vi "Add Files.vi"(8 "error in (no error)":errorcluster, 9 "Results":map{path, string}(c390), 10 "Files":set{path}(c389), 11 "File Tree In":refnum<class "File Tree.lvclass">) -> (0 "error out":errorcluster, 3 "File Tree Out":refnum<class "File Tree.lvclass">)   [LabVIEW 2020, in "File Tree.lvclass"]
uses:
  File Tree.lvclass
  File Tree.lvclass/File Tree.ctl
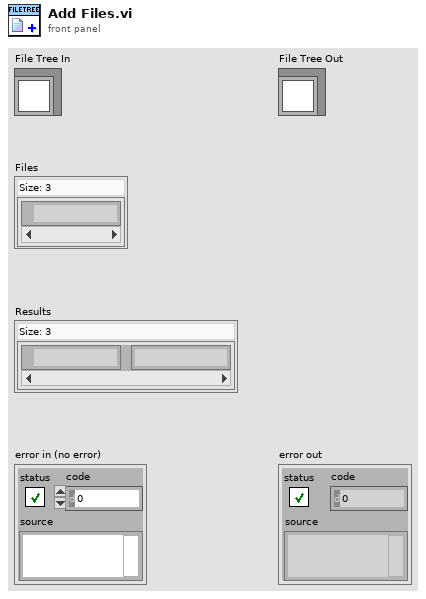
[diagram p1: front panel]
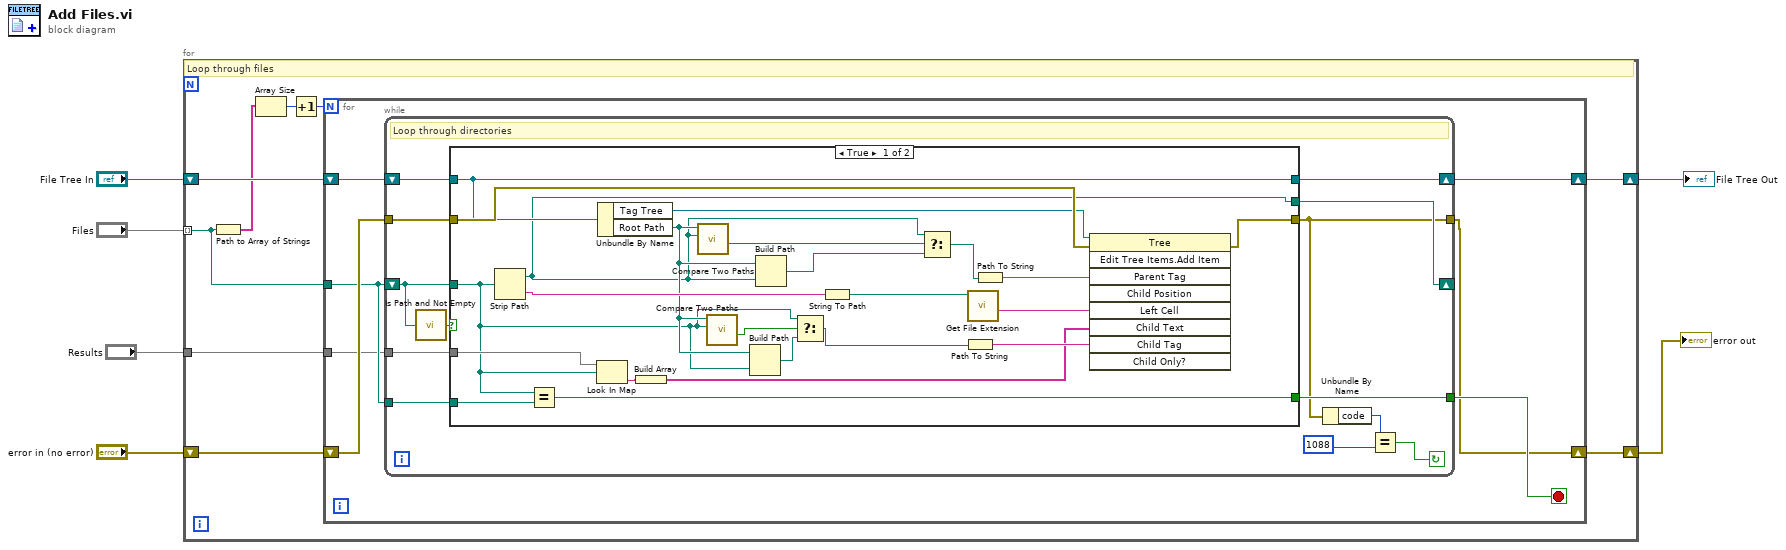
[diagram p0: block diagram]
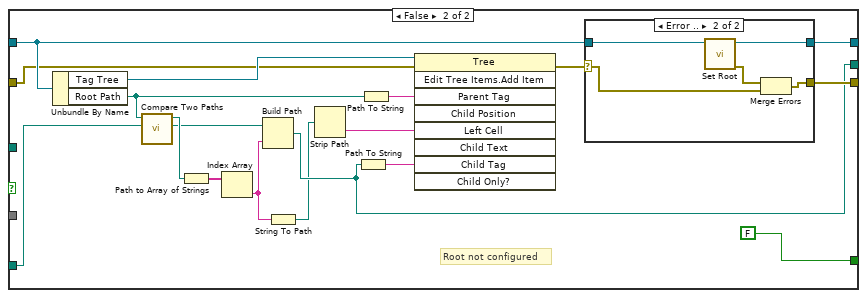
[diagram p2: hidden frame]
diagram:
  n1 = for {
    shift-right: [w15] -> w5
    shift-left: "File Tree In" -> [w14]
    shift-right: [w11] -> w6
    shift-left: "error in (no error)" -> [w12]
    tunnel: "Files" -> [w13] mode=indexing
    tunnel: "Results" -> [w7]
    # "Loop through files"
    n2 = Path to Array of Strings(0:w13) -> (2:w10:string[])  [unwired: 1 out]
    n3 = Array Size(array=w10) -> (size(s)=w9:i32)
    n4 = Increment(x=w9) -> (x+1=w8:i32)
    n5 = for {
      N: w8 -> [_]
      tunnel: w13 -> [w19]
      shift-right: [w22] -> w15
      shift-left: w14 -> [w21]
      shift-right: [w17] -> w11
      shift-left: w12 -> [w20]
      tunnel: w7 -> [w16]
      stop <- w18 stop-if-true
      n6 = while {
        shift-right: [w30] -> w22
        shift-left: w21 -> [w35]
        shift-right: [w33] -> _
        shift-left: w19 -> [w32]
        tunnel: w20 -> [w34]
        tunnel: w19 -> [w29]
        tunnel: [w28] -> w18
        tunnel: [w24] -> w17
        tunnel: w16 -> [w23]
        stop <- w25 continue-if-true
        # "Loop through directories"
        n7 = call <vilib>:"Is Path and Not Empty.vi"("path"=w32) -> ("Is Path and Not Empty?"=w31:bool)  [unwired: 4 in]
        n8 = case shown="True" w31 {
          tunnel: w35 -> [w53 w73]
          tunnel: w34 -> [w55 w70]
          tunnel: [w54 w74] -> w24
          tunnel: [w42 w63] -> w33
          tunnel: w32 -> [w37 _]
          tunnel: [w53 w75] -> w30
          tunnel: w29 -> [w52 w59]
          tunnel: [w51 FALSE] -> w28
          tunnel: w23 -> [w38 _]
          frame True {
            n9 = Strip Path(path=w37) -> (stripped path=w42:path, name=w57:string)
            n10 = Equal?(x=w37, y=w52) -> (x = y?=w51:bool)
            n11 = Look In Map(map=w38, key=w37) -> (value=w39:string)  [unwired: 1 in, 1 out]
            n12 = Unbundle By Name(w53) -> ("Tag Tree"=w43:refnum<vi>, "Root Path"=w45:path)
            n13 = Build Array(w39) -> (w36:string[])
            n14 = call <vilib>:"Compare Two Paths.vi"("Path 2"=w42, "Path 1"=w45) -> ("Path 2 Relative to Path 1?"=w50:bool)  [unwired: 6 in, 3 out]
            n15 = call <vilib>:"Compare Two Paths.vi"("Path 2"=w37, "Path 1"=w45) -> ("Path 2 Relative to Path 1?"=w49:bool)  [unwired: 6 in, 3 out]
            n16 = Build Path(base path=w45, name or relative path=w37) -> (appended path=w44:path)
            n17 = Build Path(base path=w45, name or relative path=w42) -> (appended path=w46:path)
            n18 = Select(t=w37, s=w49, f=w44) -> (s? t:f=w48:path)
            n19 = String To Path(string=w57) -> (path=w40:path)
            n20 = Select(t=w42, s=w50, f=w46) -> (s? t:f=w47:path)
            n21 = Path To String(path=w48) -> (string=w56:string)
            n22 = call <vilib>:"Get File Extension.vi"("file"=w40) -> ("filename without extension"=w41:string)  [unwired: 6 in, 4 out]
            n23 = Path To String(path=w47) -> (string=w58:string)
            n24 = invoke on="Invoke Node" class="Tree" method="Edit Tree Items.Add Item"(reference=w43, error in=w55, "Parent Tag"=w58, "Left Cell"=w41, "Child Text"=w36, "Child Tag"=w56) -> (error out=w54:errorcluster)  [unwired: 3 in, 8 out]
          }
          frame False {
            # "Root not configured"
            n25 = Unbundle By Name(w73) -> ("Tag Tree"=w72:refnum<vi>, "Root Path"=w67:path)
            n26 = call <vilib>:"Compare Two Paths.vi"("Path 2"=w59, "Path 1"=w67) -> ("Common Path"=w65:path, "Relative Path from 1 to 2"=w66:path)  [unwired: 6 in, 2 out]
            n27 = Path to Array of Strings(0:w66) -> (2:w64:string[])  [unwired: 1 out]
            n28 = Index Array(array=w64) -> (element=w62:string)  [unwired: 1 in]
            n29 = Build Path(base path=w65, name or relative path=w62) -> (appended path=w63:path)
            n30 = String To Path(string=w62) -> (path=w61:path)
            n31 = Strip Path(path=w61) -> (name=w60:string)  [unwired: 1 out]
            n32 = Path To String(path=w63) -> (string=w68:string)
            n33 = Path To String(path=w67) -> (string=w69:string)
            n34 = invoke on="Invoke Node" class="Tree" method="Edit Tree Items.Add Item"(reference=w72, error in=w70, "Parent Tag"=w69, "Left Cell"=w60, "Child Tag"=w68) -> (error out=w71:errorcluster)  [unwired: 4 in, 8 out]
            n35 = case shown="Error .." w71 {
              selector: w71 -> [w77 w79]
              tunnel: [w78 w83] -> w75
              tunnel: [w77 w80] -> w74
              tunnel: w73 -> [w78 w81]
              frame No Error {
              }
              frame Error {
                n36 = call "Set Root.vi"("File Tree In"=w81) -> ("error out"=w82:errorcluster, "File Tree Out"=w83:refnum<class "File Tree.lvclass">)  [unwired: 9 in]
                n37 = Merge Errors(w82, w79) -> (w80:errorcluster)
              }
            }
          }
        }
        n38 = Unbundle By Name(w24) -> ("code"=w27:i32)
        n39 = Equal?(x=w27, y=1088) -> (x = y?=w25:bool)
      }
    }
  }
  "error out" <- w6
  "File Tree Out" <- w5
